vi "analyseTemperature.vi"(8 "error in (no error)":errorcluster, 11 "TemperatureAnalyser in":refnum<class "TemperatureAnalyser.lvclass">) -> (0 "error out":errorcluster, 3 "TemperatureAnalyser out":refnum<class "TemperatureAnalyser.lvclass">)   [LabVIEW 2011, in "Tools.lvlib" / "Imaging.lvlib" / "TemperatureAnalyser.lvclass"]
uses:
  TemperatureAnalyser.lvclass
  Filing/FileNeologist/FileNeologist.lvclass
  Filing/FileSystem/FileSystem.lvclass
  ImageAnalyser.lvclass
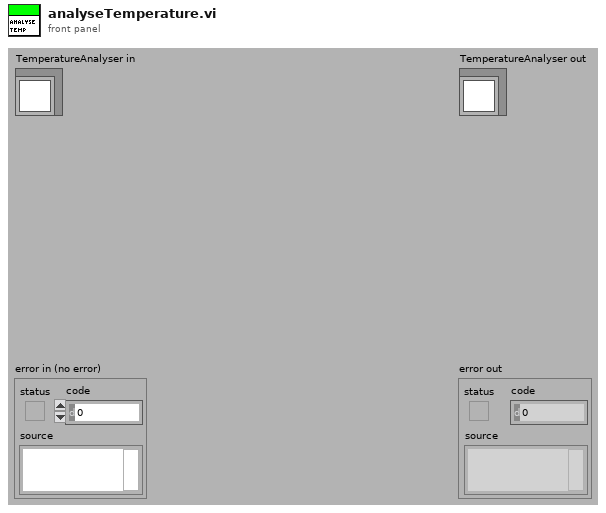
[diagram p1: front panel]
types:
  T1 = cluster{"Name":string, "Results":dbl[], "AnalysisType":string}
  T2 = cluster{"Name":string, "Results":dbl[], "AnalysisType":string}[]
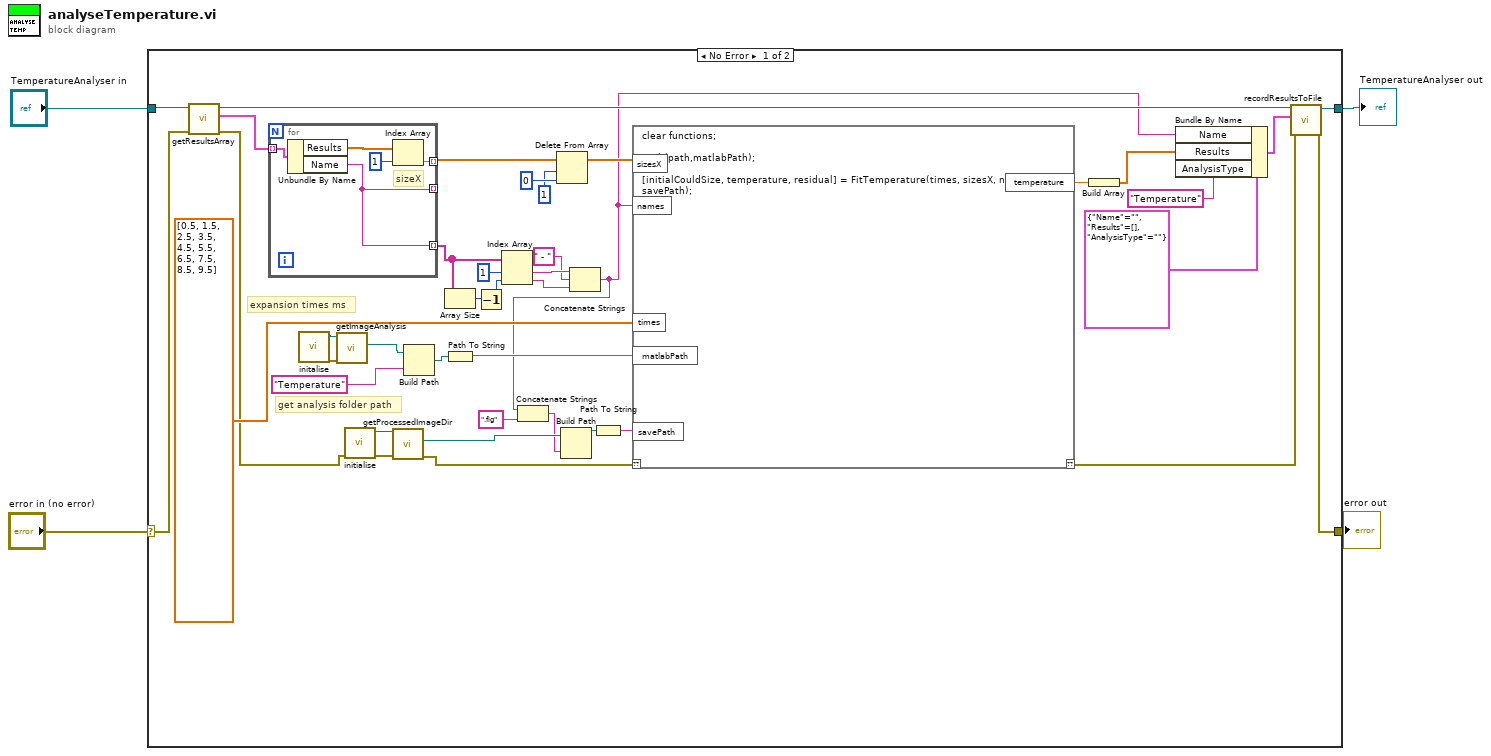
[diagram p0: block diagram]
diagram:
  n1 = case shown="No Error" "error in (no error)" {
    selector: "error in (no error)" -> [w35 w51]
    tunnel: [w26 w51] -> w3
    tunnel: [w34 w50] -> w1
    tunnel: "TemperatureAnalyser in" -> [w37 w50]
    frame No Error {
      # "get analysis folder path"
      # "expansion times ms"
      n2 = call "getResultsArray.vi"("error in (no error)"=w35, "ImageAnalyser in"=w37) -> ("error out"=w13:errorcluster, "resultsArray"=w36:T2, "ImageAnalyser out"=w33:refnum<class "TemperatureAnalyser.lvclass">)  [unwired: 7 in]
      n3 = for {
        tunnel: w36 -> [w49] mode=indexing
        tunnel: [w46] -> w24 mode=indexing
        tunnel: [w45] -> _ mode=indexing
        tunnel: [w45] -> w5 mode=indexing
        # "sizeX"
        n4 = Unbundle By Name(w49) -> ("Results"=w48:dbl[], "Name"=w45:string)
        n5 = Index Array(array=w48, index=1) -> (element=w46:dbl)
      }
      n6 = call "initalise.vi"() -> ("error out"=w42:errorcluster, "FileSystem out"=w43:refnum<class "FileSystem.lvclass">)  [unwired: 10 in]
      n7 = call "getImageAnalysis.vi"("error in (no error)"=w42, "FileSystem in"=w43) -> ("ImageAnalysis"=w41:path)  [unwired: 7 in, 2 out]
      n8 = call "initialise.vi"("error in (no error)"=w13) -> ("error out"=w16:errorcluster, "FileNeologist out"=w17:refnum<class "FileNeologist.lvclass">)  [unwired: 9 in]
      n9 = call-dynamic "getProcessedImageDir.vi"("error in (no error)"=w16, "FileNeologist in"=w17) -> ("error out"=w12:errorcluster, "Path"=w15:path)  [unwired: 7 in, 1 out]
      n10 = Build Path(base path=w41, name or relative path="Temperature") -> (appended path=w39:path)
      n11 = Array Size(array=w5) -> (size(s)=w7:i32)
      n12 = Path To String(path=w39) -> (string=w38:string)
      n13 = Decrement(x=w7) -> (x-1=w6:i32)
      n14 = Index Array(array=w5, index #1=1, index #2=w6) -> (element #1=w20:string, element #2=w19:string)
      n15 = Delete From Array(array=w24, length=1, index=0) -> (array with subset deleted=w25:dbl[])  [unwired: 1 out]
      n16 = Concatenate Strings(w20, " - ", w19) -> (w10:string)
      n17 = Concatenate Strings(w10, ".fig") -> (w11:string)
      n18 = Build Path(base path=w15, name or relative path=w11) -> (appended path=w14:path)
      n19 = Path To String(path=w14) -> (string=w8:string)
      n20 = script code="clear functions;\n\npath(path,matlabPath);\n\n[initialCouldSize, temperature, residual] = FitTemperature(times, sizesX, names, savePath);"("??"=w12, "sizesX"=w25, "times"=dbl[] [0.5, 1.5, 2.5, 3.5, 4.5, 5.5, 6.5, 7.5, 8.5, 9.5], "matlabPath"=w38, "names"=w10, "savePath"=w8) -> ("??"=w27:errorcluster, "temperature"=w32:dbl)
      n21 = Build Array(w32) -> (w29:dbl[])
      n22 = Bundle By Name(cluster=T1 {"Name"="", "Results"=[], "AnalysisType"=""} ("output cluster"), "Name"=w10, "Results"=w29, "AnalysisType"="Temperature") -> (w30:T1)
      n23 = call-dynamic "recordResultsToFile.vi"("error in (no error)"=w27, "Results"=w30, "ImageAnalyser in"=w33) -> ("error out"=w26:errorcluster, "ImageAnalyser out"=w34:refnum<class "TemperatureAnalyser.lvclass">)  [unwired: 7 in]
    }
    frame Error {
    }
  }
  "error out" <- w3
  "TemperatureAnalyser out" <- w1
